vi "AutoDelay.vi"(8 "Command Info In":T1, 9 "error in (no error)":errorcluster, 11 "Seconds to wait":dbl=0.5) -> (0 "Command Info Out":T1, 1 "error out (no error)":errorcluster)   [LabVIEW 2016]
uses:
  <vilib>/Rock Robotics/WPI/Framework/Command Status Info.ctl
  <vilib>/Rock Robotics/WPI/Framework/Completion Status.ctl
  <vilib>/Rock Robotics/WPI/Framework/Completion Notifier.ctl
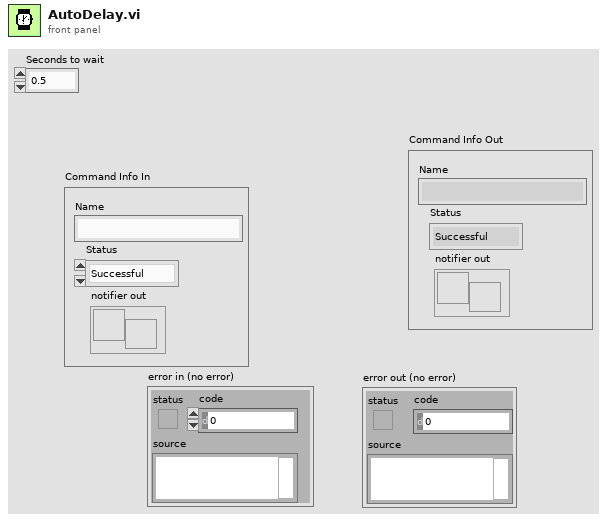
[diagram p1: front panel]
types:
  T1 = typedef "Command Status Info.ctl" = cluster{"Name":string, "Status":T2, "notifier out":T3}
  T2 = typedef "Completion Status.ctl" = enum16{"Successful", "Aborted", "Incomplete"}
  T3 = typedef "Completion Notifier.ctl" = refnum<notifier>
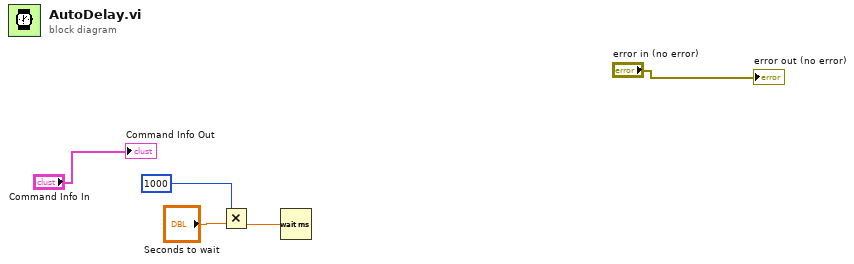
[diagram p0: block diagram]
diagram:
  n1 = Multiply(x=u32 1000, y="Seconds to wait") -> (x*y=w3:dbl)
  n2 = Wait (ms)(milliseconds to wait=w3) -> ()  [unwired: 1 out]
  "Command Info Out" <- "Command Info In"
  "error out (no error)" <- "error in (no error)"
